vi "Calculate accelerometer parameters.vi"(8 "Error In":errorcluster, 11 "Data in":sgl[](array[numeric])) -> (0 "Error Out":errorcluster, 2 "Accel Sensitivities":sgl[](array[numeric]), 3 "Accel Offset":sgl[](array[numeric]))   [LabVIEW 2016]
uses:
  Typedef/Accel FSR.ctl
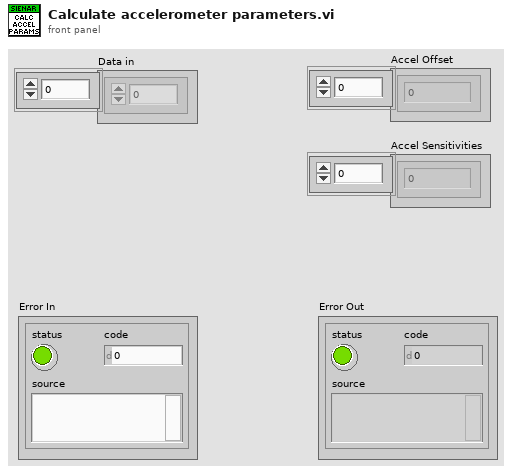
[diagram p1: front panel]
types:
  T1 = typedef "Accel FSR.ctl" = enum16{"±2g", "±4g", "±8g", "±16g"}
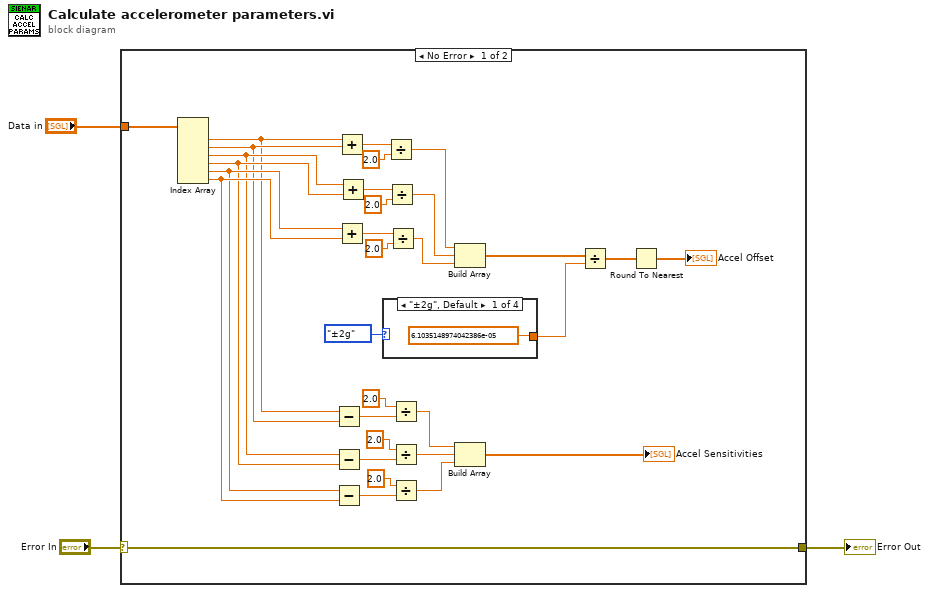
[diagram p0: block diagram]
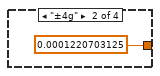
[diagram p2: hidden frame]
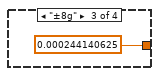
[diagram p3: hidden frame]
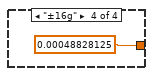
[diagram p4: hidden frame]
diagram:
  n1 = case shown="No Error" "Error In" {
    selector: "Error In" -> [w9 w40]
    tunnel: "Data in" -> [w29 _]
    tunnel: [w9 w40] -> w1
    frame No Error {
      n2 = Index Array(array=w29) -> (element #1=w30:sgl, element #2=w31:sgl, element #3=w32:sgl, element #4=w33:sgl, element #5=w34:sgl, element #6=w35:sgl)  [unwired: 6 in]
      n3 = Subtract(x=w30, y=w31) -> (x-y=w17:sgl)
      n4 = Subtract(x=w32, y=w33) -> (x-y=w15:sgl)
      n5 = Subtract(x=w34, y=w35) -> (x-y=w13:sgl)
      n6 = Add(x=w30, y=w31) -> (x+y=w27:sgl)
      n7 = Add(x=w34, y=w35) -> (x+y=w22:sgl)
      n8 = Add(x=w32, y=w33) -> (x+y=w24:sgl)
      n9 = case shown="\"±2g\", Default" Accel_FSR."±2g" ("Accel FSR") {
        tunnel: [sgl 6.103515e-05 sgl 0.00012207031 sgl 0.00024414062 sgl 0.00048828125] -> w6
        frame "±2g", Default {
        }
        frame "±4g" {
        }
        frame "±8g" {
        }
        frame "±16g" {
        }
      }
      n10 = Divide(x=w27, y=sgl 2.0) -> (x/y=w21:sgl)
      n11 = Divide(x=w24, y=sgl 2.0) -> (x/y=w20:sgl)
      n12 = Divide(x=w22, y=sgl 2.0) -> (x/y=w19:sgl)
      n13 = Divide(x=sgl 2.0 ("y"), y=w17) -> (x/y=w11:sgl)
      n14 = Divide(x=sgl 2.0 ("y"), y=w15) -> (x/y=w12:sgl)
      n15 = Divide(x=sgl 2.0 ("y"), y=w13) -> (x/y=w10:sgl)
      n16 = Build Array(w21, w20, w19) -> (w7:sgl[])
      n17 = Build Array(w11, w12, w10) -> (→"Accel Sensitivities":sgl[])
      n18 = Divide(x=w7, y=w6) -> (x/y=w5:sgl[])
      n19 = Round To Nearest(number=w5) -> (nearest integer value=→"Accel Offset":sgl[])
    }
    frame Error {
    }
  }
  "Error Out" <- w1
